vi "Test State Change.vi"(10 "Test in Progress":bool, 11 "Settings UI in":refnum<class "Settings UI.lvclass">) -> (3 "Settings UI out":refnum<class "Settings UI.lvclass">)   [LabVIEW 2020, in "Output Sequencer.lvlib" / "Settings UI.lvclass"]
uses:
  Settings UI.lvclass
  Settings UI.lvclass/Settings UI.ctl
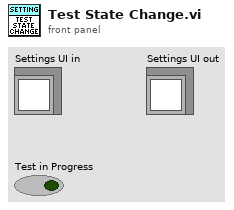
[diagram p1: front panel]
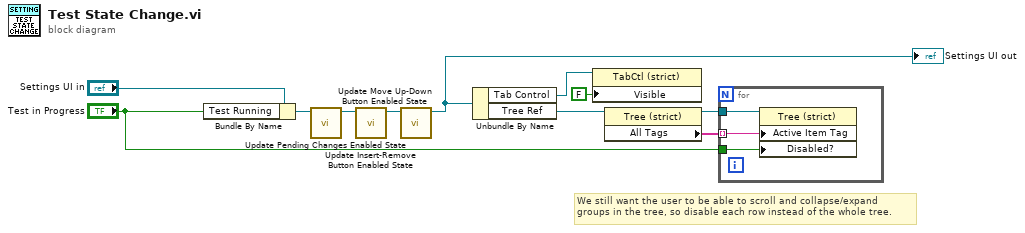
[diagram p0: block diagram]
diagram:
  # "We still want the user to be able to scroll and collapse/expand\ngroups in the tree, so disable each row instead of the whole tree."
  n1 = Bundle By Name(cluster="Settings UI in", "Test Running"="Test in Progress") -> (w4:refnum<class "Settings UI.lvclass">)
  n2 = call "Update Pending Changes Enabled State.vi"("UI Data in"=w4) -> ("UI Data out"=w5:refnum<class "Settings UI.lvclass">)  [unwired: 10 in]
  n3 = call "Update Insert-Remove Button Enabled State.vi"("UI Data in"=w5) -> ("UI Data out"=w6:refnum<class "Settings UI.lvclass">)  [unwired: 10 in]
  n4 = call "Update Move Up-Down Button Enabled State.vi"("UI Data in"=w6) -> ("UI Data out"=w7:refnum<class "Settings UI.lvclass">)  [unwired: 10 in]
  "Settings UI out" <- w7
  n5 = Unbundle By Name(w7) -> ("Tab Control"=w2:refnum<vi>, "Tree Ref"=w8:refnum<vi>)
  n6 = property on="Property Node" class="TabCtl (strict)"(reference=w2, "Visible"=FALSE) -> ()  [unwired: 1 in, 2 out]
  n7 = property on="Property Node" class="Tree (strict)"(reference=w8) -> (reference out=w10:refnum<vi>, "All Tags"=w9:string[])  [unwired: 1 in, 1 out]
  n8 = for {
    tunnel: w9 -> [w14] mode=indexing
    tunnel: w10 -> [w13]
    tunnel: "Test in Progress" -> [w12]
    n9 = property on="Property Node" class="Tree (strict)"(reference=w13, "Active Item Tag"=w14, "Disabled?"=w12) -> ()  [unwired: 1 in, 2 out]
  }
